vi "storeADCMixedToArray-wang-test2.vi"(0 "String":string) -> (18 "Graph Data":T1)   [LabVIEW 2014]
uses:
  main/controls/Graph Data.ctl
  <vilib>/Utility/miscctls.llb/LVAnnotationListTypeDef.ctl
  <vilib>/Utility/miscctls.llb/LVCursorListTypeDef.ctl
panel:
  out "CH 7":i32[](array[numeric])
  out "CH 6":i32[](array[numeric])
  out "CH 5":i32[](array[numeric])
  out "CH 4":i32[](array[numeric])
  out "CH 3":i32[](array[numeric])
  out "CH2":i32[](array[numeric])
  out "CH1":i32[](array[numeric])
  out "CH0":i32[](array[numeric])
  out "channel":u8[](array[numeric])
  out "dataADCarray":i32[](array[numeric])
  out "Waveform":waveform(dbl)
  out "Graph":waveform(i32)[](graph)
  out "Numeric 2":i32
  out "Numeric":i32
  out "TotalTrigger":i32
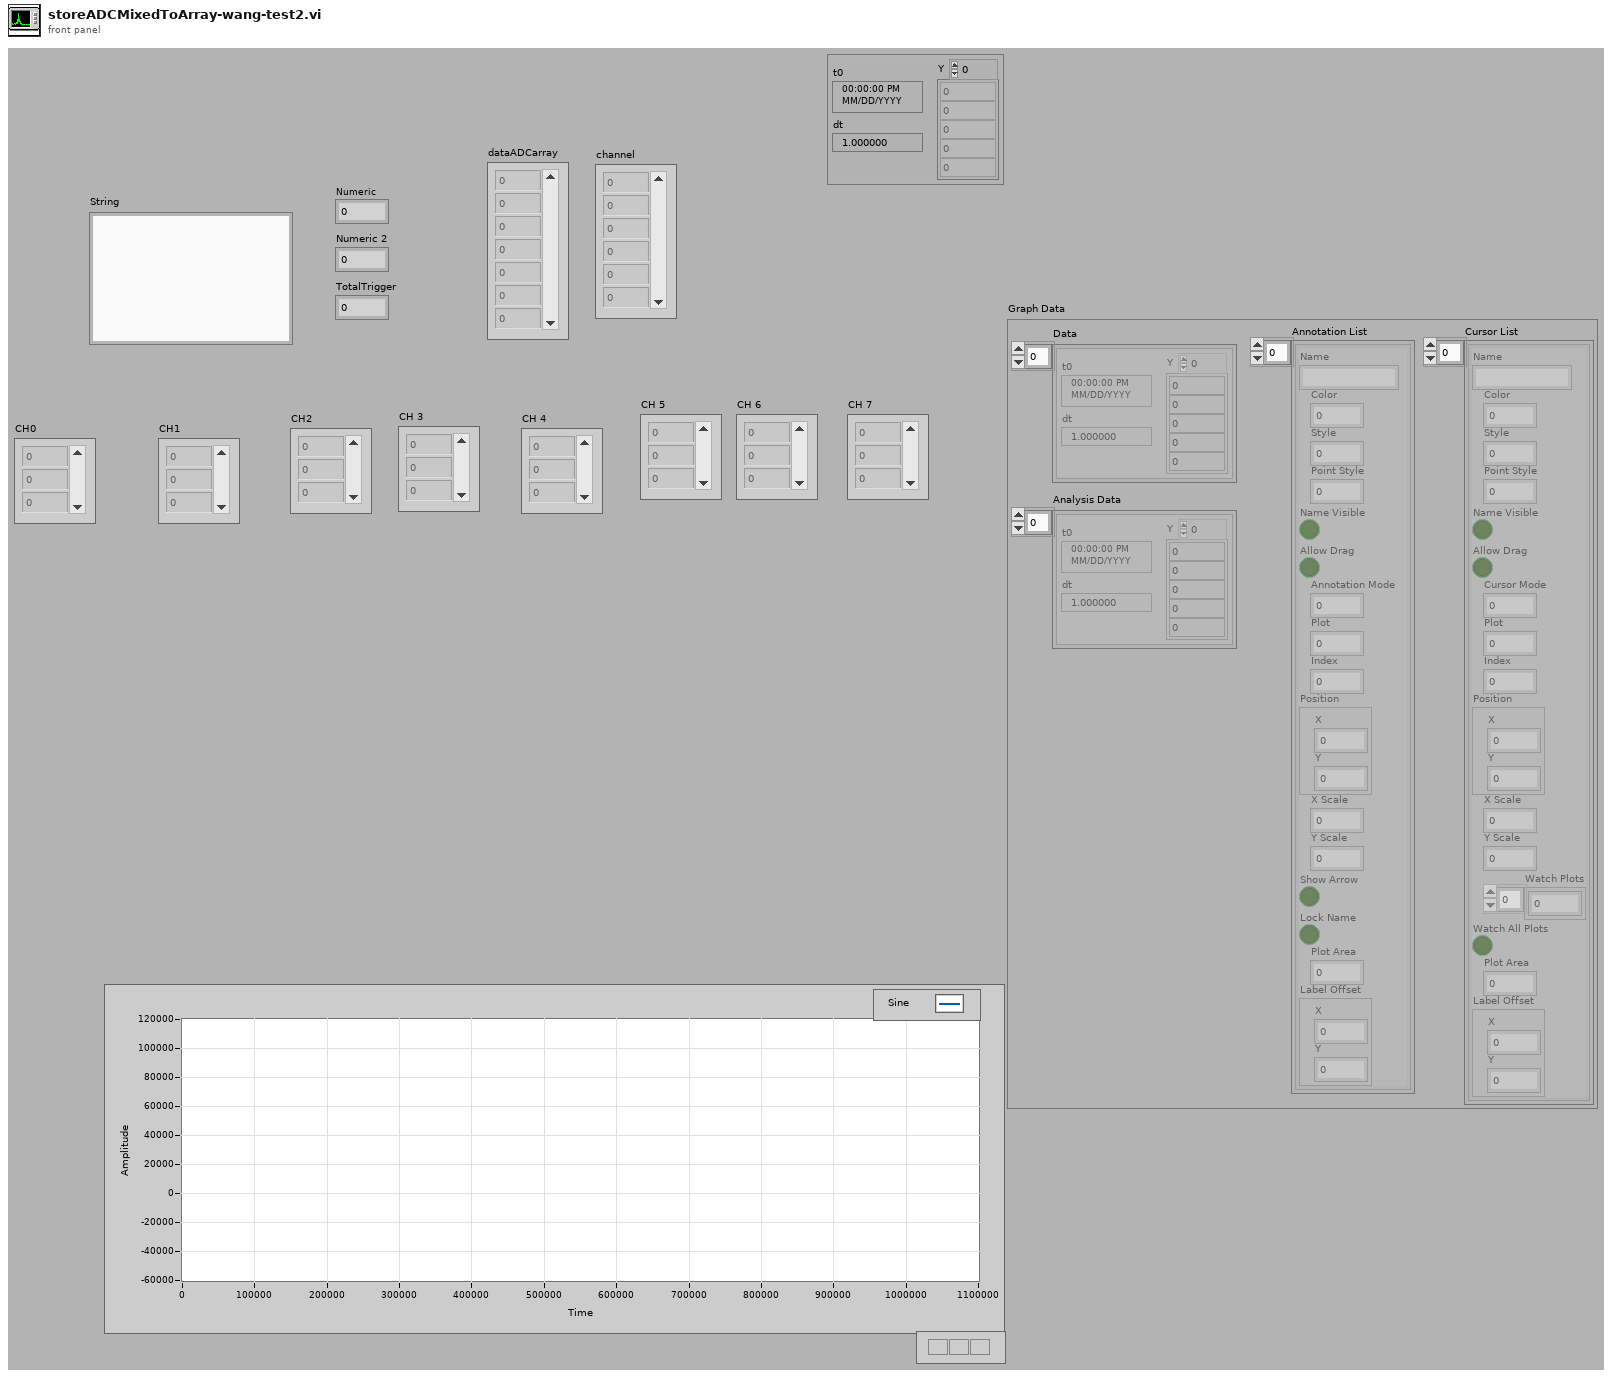
[diagram p1: front panel]
types:
  T1 = typedef "Graph Data.ctl" = cluster{"Data":waveform(dbl)[], "Annotation List":T2, "Cursor List":T3, "Analysis Data":waveform(dbl)[]}
  T2 = typedef "LVAnnotationListTypeDef.ctl" = cluster{"Name":string, "Color":u32, "Style":u8, "Point Style":u8, "Name Visible":bool, "Allow Drag":bool, "Annotation Mode":u32, "Plot":i32, "Index":i32, "Position":cluster{"X":dbl, "Y":dbl}, "X Scale":u32, "Y Scale":u32, "Show Arrow":bool, "Lock Name":bool, "Plot Area":i32, "Label Offset":cluster{"X":dbl, "Y":dbl}}[]
  T3 = typedef "LVCursorListTypeDef.ctl" = cluster{"Name":string, "Color":u32, "Style":u8, "Point Style":u8, "Name Visible":bool, "Allow Drag":bool, "Cursor Mode":u32, "Plot":i32, "Index":i32, "Position":cluster{"X":dbl, "Y":dbl}, "X Scale":u32, "Y Scale":u32, "Watch Plots":i32[], "Watch All Plots":bool, "Plot Area":i32, "Label Offset":cluster{"X":dbl, "Y":dbl}}[]
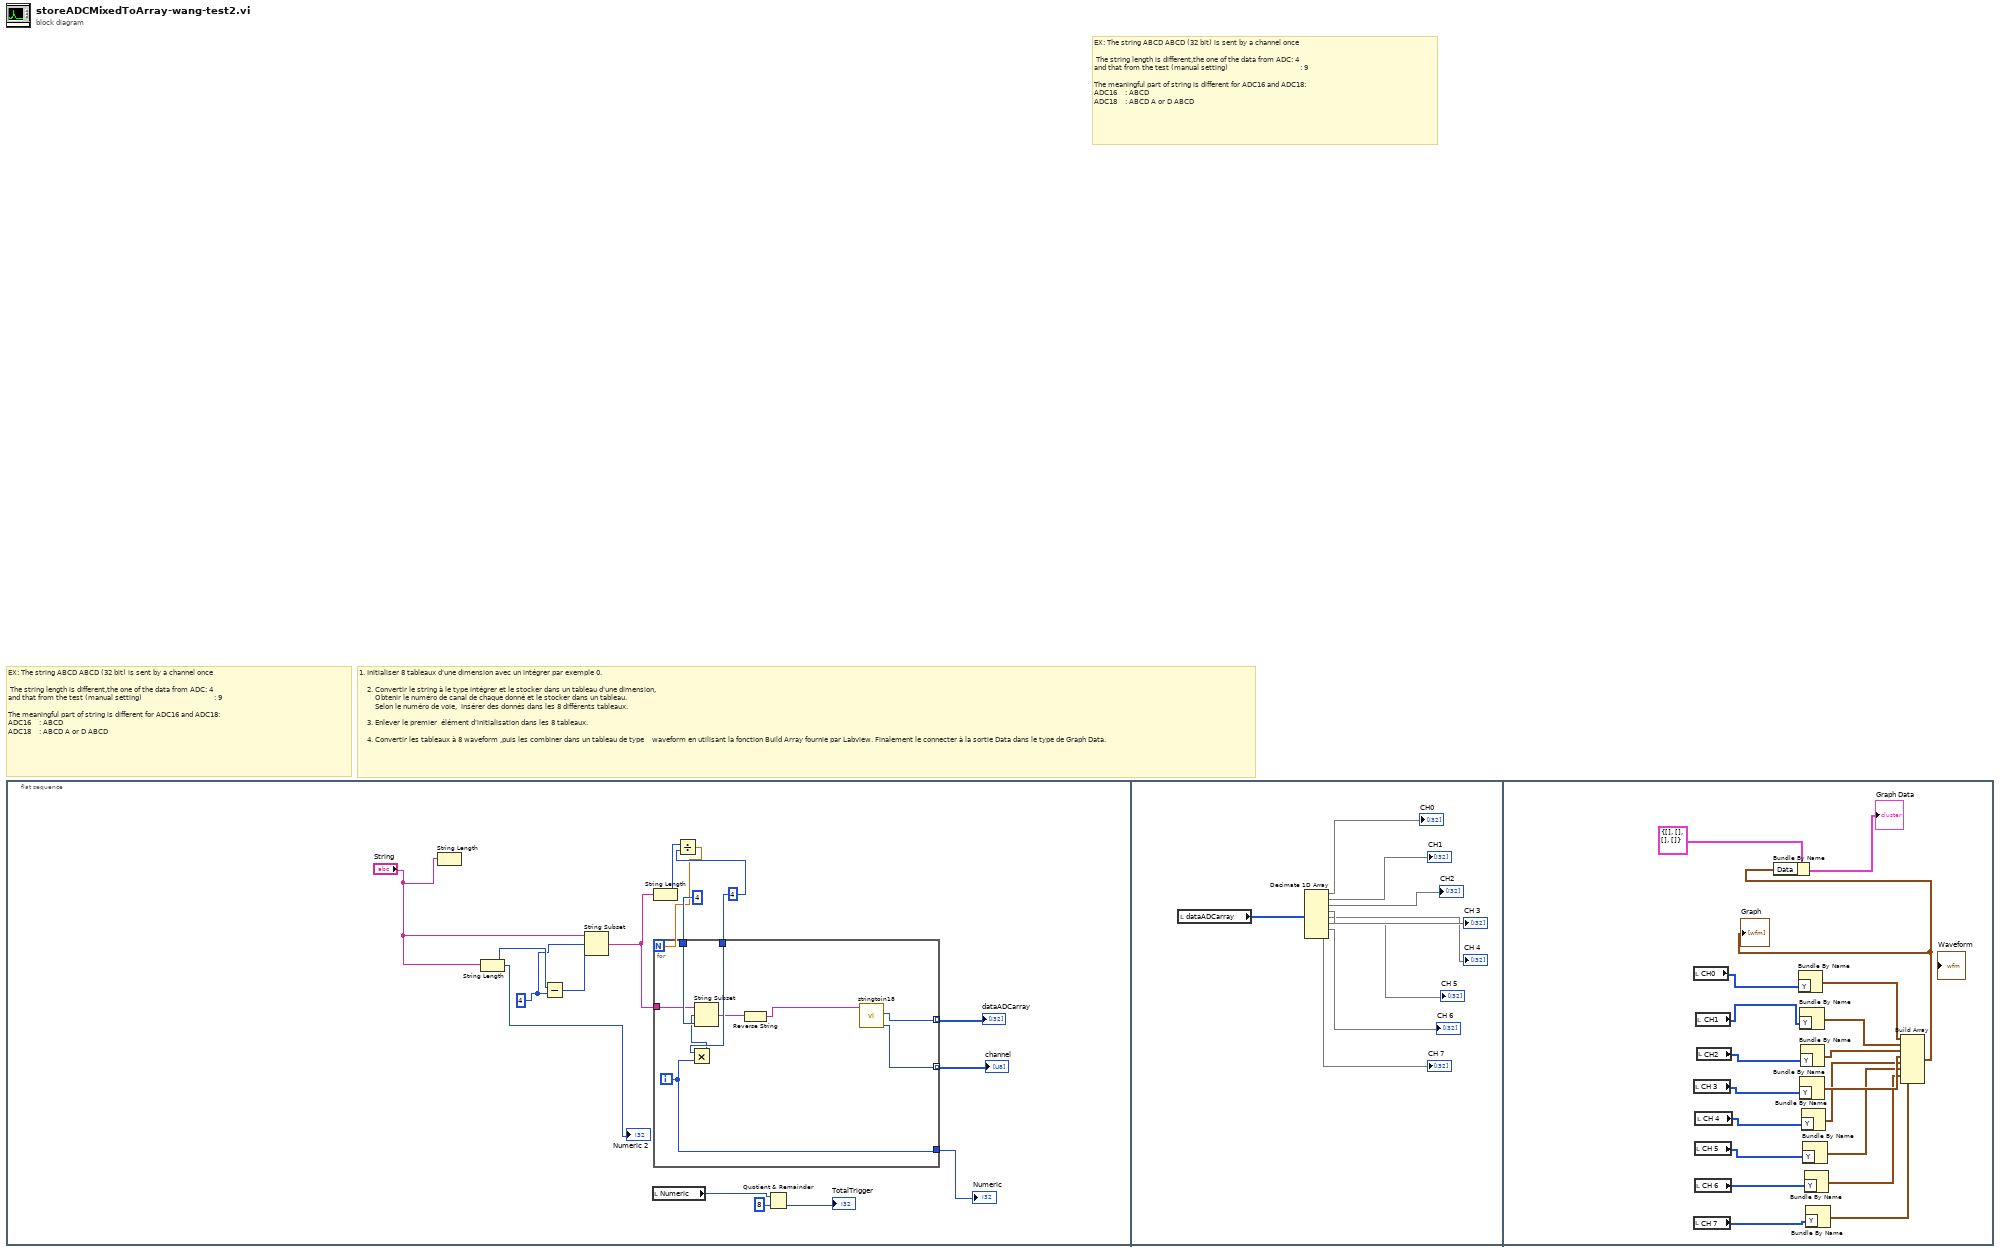
[diagram p0: block diagram]
diagram:
  # "1. Initialiser 8 tableaux d'une dimension avec un intégrer par exemple 0.\n\n    2.\tConvertir le string à le type intégrer et le stocker dans un tableau d'une dimension,\n        Obtenir le numéro de canal de chaque donné et le stocker dans un tableau.  \n        Selon le numéro de voie,  Insérer des donnés dans les 8 différents tableaux.\n\n    3. Enlever le premier  élément d'initialisation dans les 8 tableaux.\n\n    4. Convertir les tableaux à 8 waveform ,puis les combiner dans un tableau de type    waveform en utilisant la fonction Build Array fournie par Labview. Finalement le connecter à la sortie Data dans le type de Graph Data."
  # "EX: The string ABCD ABCD (32 bit) is sent by a channel once                \n\n The string length is different,the one of the data from ADC: 4\nand that from the test (manual setting)                                    : 9\n\nThe meaningful part of string is different for ADC16 and ADC18:\nADC16    : ABCD                          \nADC18    : ABCD A or D ABCD"
  # "EX: The string ABCD ABCD (32 bit) is sent by a channel once                \n\n The string length is different,the one of the data from ADC: 4\nand that from the test (manual setting)                                    : 9\n\nThe meaningful part of string is different for ADC16 and ADC18:\nADC16    : ABCD                          \nADC18    : ABCD A or D ABCD"
  n1 = flat-sequence {
    frame #0 {
      w9 = 4
      w12 = 4
      n2 = String Length(string="String") -> ()  [unwired: 1 out]
      n3 = String Length(string="String") -> (length=w15:i32)
      "Numeric 2" <- w15
      n4 = Subtract(x=w15, y=w12) -> (x-y=w13:i32)
      n5 = String Subset(string="String", offset (0)=w12, length (rest)=w13) -> (substring=w7:string)
      n6 = local read "Numeric"() -> (w4:i32)
      n7 = String Length(string=w7) -> (length=w10:i32)
      n8 = Divide(x=w10, y=w9) -> (x/y=w8:dbl)
      n9 = for {
        N: w8 -> [_]
        tunnel: 4 -> [w24]
        tunnel: w9 -> [w23]
        tunnel: [w19] -> w14
        tunnel: w7 -> [w20]
        tunnel: [w17] -> w2 mode=indexing
        tunnel: [w16] -> w1 mode=indexing
        i -> [w19]
        n10 = Multiply(x=w23, y=w19) -> (x*y=w22:i32)
        n11 = String Subset(string=w20, offset (0)=w22, length (rest)=w24) -> (substring=w21:string)
        n12 = Reverse String(1:w21) -> (0:w18:string)
        n13 = call "stringtoin18.vi"("input_string"=w18) -> ("channel"=w16:u8, "outputComplemented_int"=w17:i32)  [unwired: 7 in, 2 out]
      }
      "Numeric" <- w14
      "dataADCarray" <- w2
      "channel" <- w1
      n14 = Quotient & Remainder(x=w4, y=8) -> (floor(x/y)=→"TotalTrigger":i32)  [unwired: 1 out]
    }
    frame #1 {
      n15 = local read "dataADCarray"() -> (w33:i32[])
      n16 = Decimate 1D Array(w33) -> (→"CH0":i32[], →"CH1":i32[], →"CH2":i32[], →"CH 3":i32[], →"CH 4":i32[], →"CH 5":i32[], →"CH 6":i32[], →"CH 7":i32[])
    }
    frame #2 {
      n17 = local read "CH0"() -> (w52:i32[])
      n18 = local read "CH 3"() -> (w44:i32[])
      n19 = local read "CH 7"() -> (w48:i32[])
      n20 = local read "CH 5"() -> (w46:i32[])
      n21 = local read "CH 6"() -> (w47:i32[])
      n22 = local read "CH 4"() -> (w45:i32[])
      n23 = local read "CH1"() -> (w50:i32[])
      n24 = local read "CH2"() -> (w43:i32[])
      n25 = Bundle By Name("Y"=w52) -> (w51:waveform(i32))  [unwired: 1 in]
      n26 = Bundle By Name("Y"=w50) -> (w49:waveform(i32))  [unwired: 1 in]
      n27 = Bundle By Name("Y"=w44) -> (w41:waveform(i32))  [unwired: 1 in]
      n28 = Bundle By Name("Y"=w43) -> (w42:waveform(i32))  [unwired: 1 in]
      n29 = Bundle By Name("Y"=w45) -> (w37:waveform(i32))  [unwired: 1 in]
      n30 = Bundle By Name("Y"=w46) -> (w40:waveform(i32))  [unwired: 1 in]
      n31 = Bundle By Name("Y"=w47) -> (w39:waveform(i32))  [unwired: 1 in]
      n32 = Bundle By Name("Y"=w48) -> (w38:waveform(i32))  [unwired: 1 in]
      n33 = Build Array(w51, w49, w42, w41, w37, w40, w39, w38) -> (w36:waveform(i32)[])
      "Graph" <- w36
      n34 = Bundle By Name(cluster=T1 {"Data"=[], "Annotation List"=[], "Cursor List"=[], "Analysis Data"=[]} ("Graph Data"), "Data"=w36) -> (→"Graph Data":T1)
    }
  }
